vi "PWMAutoDirection.vi"(7 "Motor Select":i8, 8 "Error in":errorcluster, 10 "PWM Frequency":dbl=100.0, 11 "DutyCycle":dbl) -> (0 "error out":errorcluster)   [LabVIEW 2014]
uses:
  <vilib>/myRIO/Instrument Drivers/Onboard IO/DIO/typedefs/DIO Reference.ctl
  <vilib>/myRIO/Common/Instrument Driver Framework/Utilities/typedefs/myRIO Generic Hardware Reference.ctl
  <vilib>/myRIO/Common/Instrument Driver Framework/Utilities/typedefs/Hardware Version Enum.ctl
  <vilib>/myRIO/Common/Instrument Driver Framework/Utilities/typedefs/myRIO v1.0 Reference.ctl
  <vilib>/myRIO/Common/Instrument Driver Framework/Utilities/typedefs/Generic FPGA Reference.ctl
  <vilib>/myRIO/Common/Instrument Driver Framework/myRIO v1.0/DIO/typedefs/DIO Channels List.ctl
  <vilib>/myRIO/Common/Instrument Driver Framework/myRIO v1.0/DIO/typedefs/DIO Channels Enum.ctl
  <vilib>/userdefined/High Color/nirio_resource_hc.ctl
  <vilib>/myRIO/Instrument Drivers/Onboard IO/PWM/typedefs/PWM Reference.ctl
  <vilib>/myRIO/Common/Instrument Driver Framework/myRIO v1.0/PWM/typedefs/PWM Channels Enum.ctl
  <vilib>/myRIO/Instrument Drivers/Onboard IO/PWM/typedefs/PWM Configuration.ctl
  <vilib>/myRIO/Common/Instrument Driver Framework/Utilities/vis/Is FPGA Ref Available.vi
  <vilib>/myRIO/Common/Instrument Driver Framework/myRIO v1.0/DIO/vis/myRIO v1.1 Open DIO.vi
  <vilib>/myRIO/Instrument Drivers/Onboard IO/DIO/vis/Write.vi
  <vilib>/myRIO/Common/Instrument Driver Framework/myRIO v1.0/PWM/vis/myRIO v1.1 Open PWM.vi
  <vilib>/myRIO/Instrument Drivers/Onboard IO/PWM/vis/Set Duty Cycle and Frequency.vi
  <vilib>/myRIO/Common/Instrument Driver Framework/Utilities/vis/Validate Channels.vi
  <vilib>/myRIO/Common/Instrument Driver Framework/myRIO v1.0/DIO/vis/myRIO v1.0 Reserve DIO.vi
  <vilib>/myRIO/Common/Instrument Driver Framework/myRIO v1.0/PWM/vis/myRIO v1.0 Reserve PWM.vi
  <vilib>/myRIO/Common/Instrument Driver Framework/myRIO v1.0/Resource Manager/vis/myRIO v1.0 Reserve Channel List.vi
  <vilib>/myRIO/Common/Instrument Driver Framework/myRIO v1.0/DIO/vis/myRIO v1.0 Build MUX Configuration DIO.vi
  <vilib>/myRIO/Common/Instrument Driver Framework/myRIO v1.0/PWM/vis/myRIO v1.0 Build MUX Configuration PWM.vi
  <vilib>/myRIO/Common/Instrument Driver Framework/myRIO v1.0/Resource Manager/vis/myRIO v1.0 Reserve Channel.vi
  <vilib>/myRIO/Common/Instrument Driver Framework/myRIO v1.0/Resource Manager/vis/myRIO v1.0 Unreserve Channel.vi
  <vilib>/myRIO/Common/Instrument Driver Framework/myRIO v1.0/Resource Manager/vis/myRIO v1.0 Create Configuration List.vi
  <vilib>/myRIO/Common/Instrument Driver Framework/myRIO v1.0/Resource Manager/vis/myRIO v1.0 Build Mutex Name.vi
  <vilib>/Utility/VariantDataType/GetNumericInfo.vi
  <vilib>/Utility/error.llb/Error Cluster From Error Code.vi
  <vilib>/myRIO/Common/Instrument Driver Framework/myRIO v1.0/myRIO v1.1 Open.vi
  <vilib>/myRIO/Common/Instrument Driver Framework/Utilities/vis/IO Manager.vi
  <vilib>/myRIO/Common/Instrument Driver Framework/Utilities/vis/Configuration Manager.vi
  <vilib>/myRIO/Common/Instrument Driver Framework/myRIO v1.0/Resource Manager/vis/myRIO v1.0 Configure IO.vi
  <vilib>/myRIO/Common/Instrument Driver Framework/myRIO v1.0/myRIO v1.0 Close.vi
  <vilib>/myRIO/Common/Instrument Driver Framework/myRIO v1.0/DIO/vis/myRIO v1.0 Write DIO.vi
  <vilib>/myRIO/Common/Instrument Driver Framework/myRIO v1.0/PWM/vis/myRIO v1.0 Write PWM.vi
  <vilib>/myRIO/Express VI/Onboard IO/DO/DO Express VI.xnode
  <vilib>/myRIO/Instrument Drivers/Onboard IO/DIO/vis/myRIO DIO Open.xnode
  <vilib>/myRIO/Express VI/Onboard IO/PWM/PWM Express VI.xnode
  <vilib>/myRIO/Instrument Drivers/Onboard IO/PWM/vis/myRIO PWM Open.xnode
  <vilib>/myRIO/Instrument Drivers/Onboard IO/DIO/DIO.lvlib
  <vilib>/myRIO/Instrument Drivers/Onboard IO/PWM/PWM.lvlib
panel:
  # "This VI will change the direction automatically for a given duty cycle between \n-1 and 1. Negative values will make the motors turn backwards."
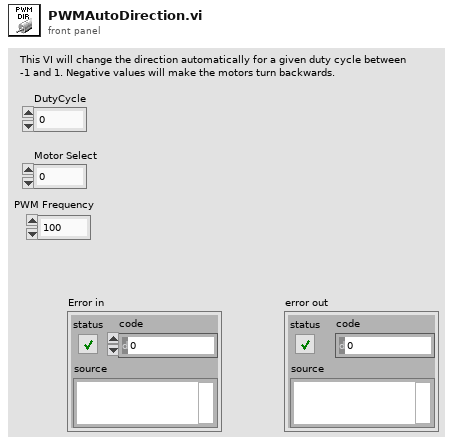
[diagram p1: front panel]
types:
  T1 = typedef "PWM.lvlib/PWM Reference.ctl" = cluster{"myRIO Reference":T2, "PWM Channels Enum":T6, "PWM Configuration":T7}
  T2 = typedef "myRIO Generic Hardware Reference.ctl" = cluster{"myRIO Model":T3, "myRIO Hardware Reference":T4}
  T3 = typedef "Hardware Version Enum.ctl" = enum16{"Unknown", "myRIO-1900", "myRIO-1950"}
  T4 = typedef "myRIO v1.0 Reference.ctl" = cluster{"Generic FPGA Reference":T5, "Allow multiple opens":bool}
  T5 = typedef "Generic FPGA Reference.ctl" = refnum<k20>
  T6 = typedef "PWM Channels Enum.ctl" = enum16{"Not Connected", "C/PWM0", "C/PWM1", "A/PWM0", "A/PWM1", "A/PWM2", "B/PWM0", "B/PWM1", "B/PWM2"}
  T7 = typedef "PWM.lvlib/PWM Configuration.ctl" = cluster{"Frequency":dbl, "Duty Cycle":dbl}
  T8 = typedef "nirio_resource_hc.ctl" = tag
  T9 = typedef "DIO.lvlib/DIO Reference.ctl" = cluster{"myRIO Reference":T2, "DIO Channels List":T10}
  T10 = typedef "DIO Channels List.ctl" = T11[]
  T11 = typedef "DIO Channels Enum.ctl" = enum16{"Not Connected", "C/DIO0", "C/DIO1", "C/DIO2", "C/DIO3", "C/DIO4", "C/DIO5", "C/DIO6", "C/DIO7", "A/DIO0", "A/DIO1", "A/DIO2", "A/DIO3", "A/DIO4", "A/DIO5", "A/DIO6", "A/DIO7", "A/DIO8", "A/DIO9", "A/DIO10", "A/DIO11", "A/DIO12", "A/DIO13", "A/DIO14", "A/DIO15", "B/DIO0", "B/DIO1", "B/DIO2", "B/DIO3", "B/DIO4", "B/DIO5", "B/DIO6", "B/DIO7", "B/DIO8", "B/DIO9", "B/DIO10", "B/DIO11", "B/DIO12", "B/DIO13", "B/DIO14", "B/DIO15", "LED0", "LED1", "LED2", "LED3", "Button0"}
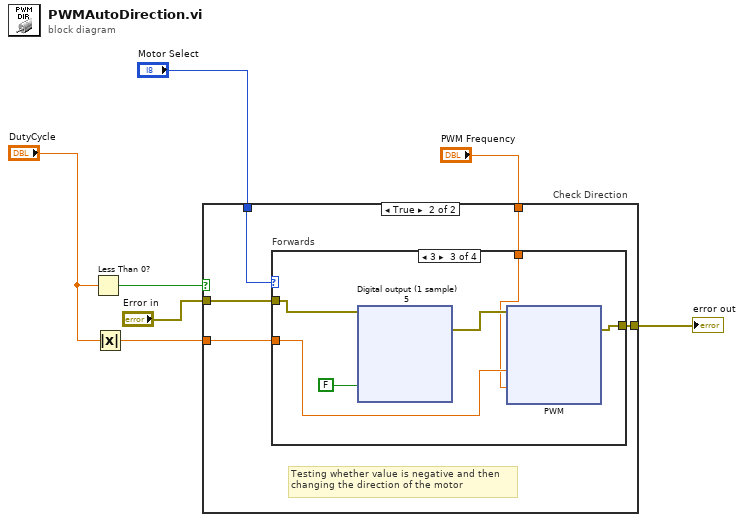
[diagram p0: block diagram]
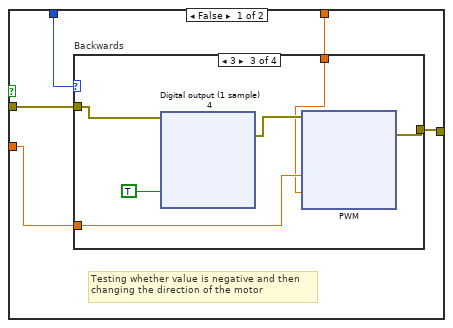
[diagram p2: hidden frame]
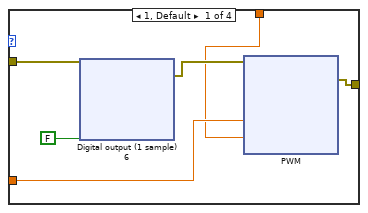
[diagram p3: hidden frame]
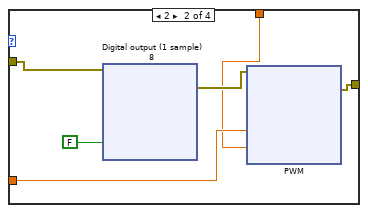
[diagram p4: hidden frame]
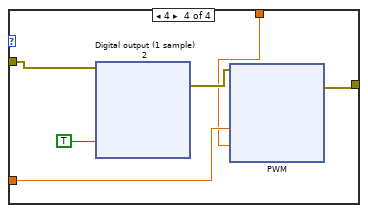
[diagram p5: hidden frame]
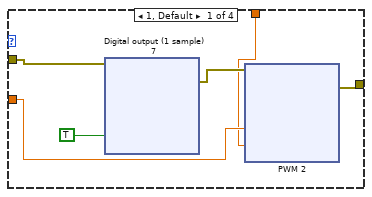
[diagram p6: hidden frame]
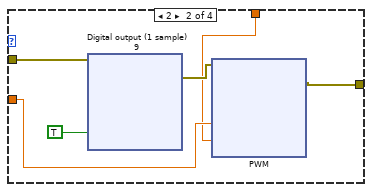
[diagram p7: hidden frame]
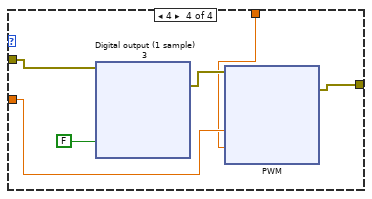
[diagram p8: hidden frame]
diagram:
  n1 = Less Than 0?(x="DutyCycle") -> (x < 0?=w4:bool)
  n2 = Absolute Value(x="DutyCycle") -> (abs(x)=w5:dbl)
  n3 = case "Check Direction" shown="True" w4 {
    tunnel: "Motor Select" -> [w12 w321]
    tunnel: w5 -> [w11 w320]
    tunnel: "PWM Frequency" -> [w10 w319]
    tunnel: "Error in" -> [w9 w318]
    tunnel: [w8 w317] -> w1
    frame False {
      # "Testing whether value is negative and then\nchanging the direction of the motor"
      n4 = case "Backwards" shown="3" w12 {
        tunnel: w11 -> [w16 w90 w166 w242]
        tunnel: w10 -> [w13 w89 w165 w241]
        tunnel: w9 -> [w17 w93 w169 w245]
        tunnel: [w14 w91 w168 w244] -> w8
        frame 1, Default {
          n5 = xnode ("Digital output (1 sample) 6")("DIR1 (B/DIO6 (Pin 23))"=FALSE ("DIR4 (A/DIO7 (Pin 25)) 5"), "error in (no error)"=w17) -> ("error out"=w15:errorcluster)
          n6 = xnode "PWM"("Duty Cycle"=w16, "Frequency [Hz]"=w13, "error in (no error)"=w15) -> ("error out"=w14:errorcluster)
        }
        frame 2 {
          n7 = xnode ("Digital output (1 sample) 8")("DIR2 (B/DIO7 (Pin 25))"=FALSE ("DIR4 (A/DIO7 (Pin 25)) 7"), "error in (no error)"=w93) -> ("error out"=w92:errorcluster)
          n8 = xnode "PWM"("Duty Cycle"=w90, "Frequency [Hz]"=w89, "error in (no error)"=w92) -> ("error out"=w91:errorcluster)
        }
        frame 3 {
          n9 = xnode ("Digital output (1 sample) 4")("DIR3 (A/DIO6 (Pin 23))"=TRUE ("DIR4 (A/DIO7 (Pin 25)) 3"), "error in (no error)"=w169) -> ("error out"=w167:errorcluster)
          n10 = xnode "PWM"("Duty Cycle"=w166, "Frequency [Hz]"=w165, "error in (no error)"=w167) -> ("error out"=w168:errorcluster)
        }
        frame 4 {
          n11 = xnode ("Digital output (1 sample) 2")("DIR4 (A/DIO7 (Pin 25))"=TRUE ("DIR4 (A/DIO7 (Pin 25)) 9"), "error in (no error)"=w245) -> ("error out"=w243:errorcluster)
          n12 = xnode "PWM"("Duty Cycle"=w242, "Frequency [Hz]"=w241, "error in (no error)"=w243) -> ("error out"=w244:errorcluster)
        }
      }
    }
    frame True {
      # "Testing whether value is negative and then\nchanging the direction of the motor"
      n13 = case "Forwards" shown="3" w321 {
        tunnel: w320 -> [w323 w399 w476 w552]
        tunnel: w319 -> [w322 w398 w475 w551]
        tunnel: w318 -> [w326 w402 w478 w554]
        tunnel: [w324 w400 w474 w550] -> w317
        frame 1, Default {
          n14 = xnode ("Digital output (1 sample) 7")("DIR1 (B/DIO6 (Pin 23))"=TRUE ("DIR4 (A/DIO7 (Pin 25)) 6"), "error in (no error)"=w326) -> ("error out"=w325:errorcluster)
          n15 = xnode "PWM 2"("Duty Cycle"=w323, "Frequency [Hz]"=w322, "error in (no error)"=w325) -> ("error out"=w324:errorcluster)
        }
        frame 2 {
          n16 = xnode ("Digital output (1 sample) 9")("DIR2 (B/DIO7 (Pin 25))"=TRUE ("DIR4 (A/DIO7 (Pin 25)) 8"), "error in (no error)"=w402) -> ("error out"=w401:errorcluster)
          n17 = xnode "PWM"("Duty Cycle"=w399, "Frequency [Hz]"=w398, "error in (no error)"=w401) -> ("error out"=w400:errorcluster)
        }
        frame 3 {
          n18 = xnode ("Digital output (1 sample) 5")("DIR3 (A/DIO6 (Pin 23))"=FALSE ("DIR4 (A/DIO7 (Pin 25)) 4"), "error in (no error)"=w478) -> ("error out"=w477:errorcluster)
          n19 = xnode "PWM"("Duty Cycle"=w476, "Frequency [Hz]"=w475, "error in (no error)"=w477) -> ("error out"=w474:errorcluster)
        }
        frame 4 {
          n20 = xnode ("Digital output (1 sample) 3")("DIR4 (A/DIO7 (Pin 25))"=FALSE ("DIR4 (A/DIO7 (Pin 25)) 2"), "error in (no error)"=w554) -> ("error out"=w553:errorcluster)
          n21 = xnode "PWM"("Duty Cycle"=w552, "Frequency [Hz]"=w551, "error in (no error)"=w553) -> ("error out"=w550:errorcluster)
        }
      }
    }
  }
  "error out" <- w1
